vi "WPI_RobotDriveOpen6MotorWithVictor.vi"(0 "Rear Left Motor":T1=enum."PWM 2", 1 "Rear Left Motor Inverted":bool, 2 "Rear Right Motor Inverted":bool=TRUE, 5 "Rear Right Motor":T1, 7 "Front Left Motor":T1=enum."PWM 4", 9 "Front Right Motor":T1=enum."PWM 3", 11 "error in (no error)":errorcluster, 12 "Front Left Motor Inverted":bool, 13 "Front Right Motor Inverted":bool=TRUE) -> (4 "RobotDriveDevRef":T2={"DevStatus"={"status"=FALSE, "code"=0, "source"=""}, "Motors[]"=[], "Square Inputs"=FALSE, "Max Output"=1.0, "Isochronous"=FALSE}, 15 "error out":errorcluster)   [LabVIEW 2013]
doc: "Opens a reference to the robot drive for a four-motor robot using Victor motor controllers.\n\nThis software is licensed. Open the labview\\readme\\WPI Robotics Library Open Source License.txt file for more information."
uses:
  <vilib>/Rock Robotics/SystemInterfaces/DIO/FPGA_DIOPWMChannel.ctl
  <vilib>/Rock Robotics/WPI/RobotDrive/WPI_RobotDriveDevRef.ctl
  <vilib>/Rock Robotics/WPI/MotorControl/WPI_MotorControlDeviceRef.ctl
  <vilib>/Rock Robotics/SystemInterfaces/Typedef/FPGA_TypedefDigitalModule.ctl
  <vilib>/Rock Robotics/WPI/PWM/WPI_PWMDeadband.ctl
  <vilib>/Rock Robotics/WPI/CAN/Jaguar/SubVIs/WPI_CANJaguar_ControlMode.ctl
  <vilib>/Rock Robotics/WPI/PWM/WPI_PWMTransform_ConPane.ctl
  <vilib>/Rock Robotics/WPI/SafetyOutput/WPI_SafetyOutputConfigMenu.ctl
  <vilib>/Rock Robotics/WPI/MotorControl/WPI_MotorControlOpen Victor.vi
panel:
  in  "Mid Right Motor Inverted":bool=TRUE
  in  "Mid LeftMotor Inverted":bool
  in  "Mid Right Motor":T1=enum."PWM 5"
  in  "Mid Left Motor":T1=enum."PWM 6"
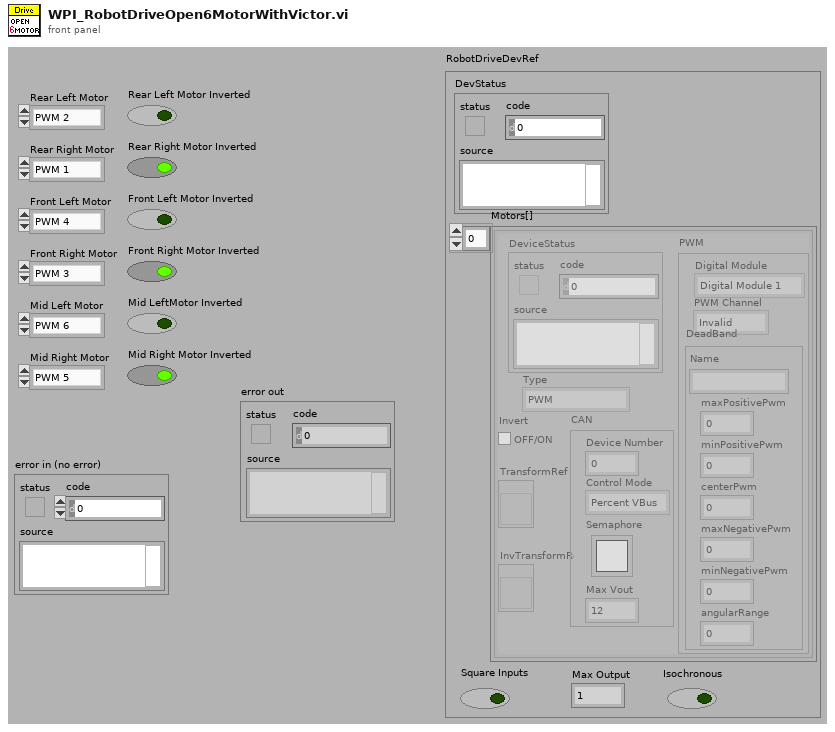
[diagram p1: front panel]
types:
  T1 = typedef "FPGA_DIOPWMChannel.ctl" = enum8{"PWM 1", "PWM 2", "PWM 3", "PWM 4", "PWM 5", "PWM 6", "PWM 7", "PWM 8", "PWM 9", "PWM 10", "Invalid"}
  T2 = typedef "WPI_RobotDriveDevRef.ctl" = cluster{"DevStatus":errorcluster, "Motors[]":T3[], "Square Inputs":bool, "Max Output":dbl, "Isochronous":bool}
  T3 = typedef "WPI_MotorControlDeviceRef.ctl" = cluster{"DeviceStatus":errorcluster, "Type":enum16{"PWM", "CAN"}, "PWM":cluster{"Digital Module":T4, "PWM Channel":T1, "DeadBand":T5}, "CAN":cluster{"Device Number":u8, "Control Mode":T6, "Semaphore":T7, "Max Vout":dbl}, "Invert":bool, "TransformRef":T8, "InvTransformRef":T8}
  T4 = typedef "FPGA_TypedefDigitalModule.ctl" = enum16{"Digital Module 1", "Digital Module 2"}
  T5 = typedef "WPI_PWMDeadband.ctl" = cluster{"Name":string, "maxPositivePwm":i32, "minPositivePwm":i32, "centerPwm":i32, "maxNegativePwm":i32, "minNegativePwm":i32, "angularRange":u16}
  T6 = typedef "WPI_CANJaguar_ControlMode.ctl" = enum8{"Percent VBus", "Current", "Speed", "Position", "Voltage"}
  T7 = typedef "Semaphore RefNum" = refnum<k1>
  T8 = typedef "WPI_PWMTransform_ConPane.ctl" = refnum<vi>
  T9 = typedef "WPI_SafetyOutputConfigMenu.ctl" = enum16{"Enable", "Disable"}
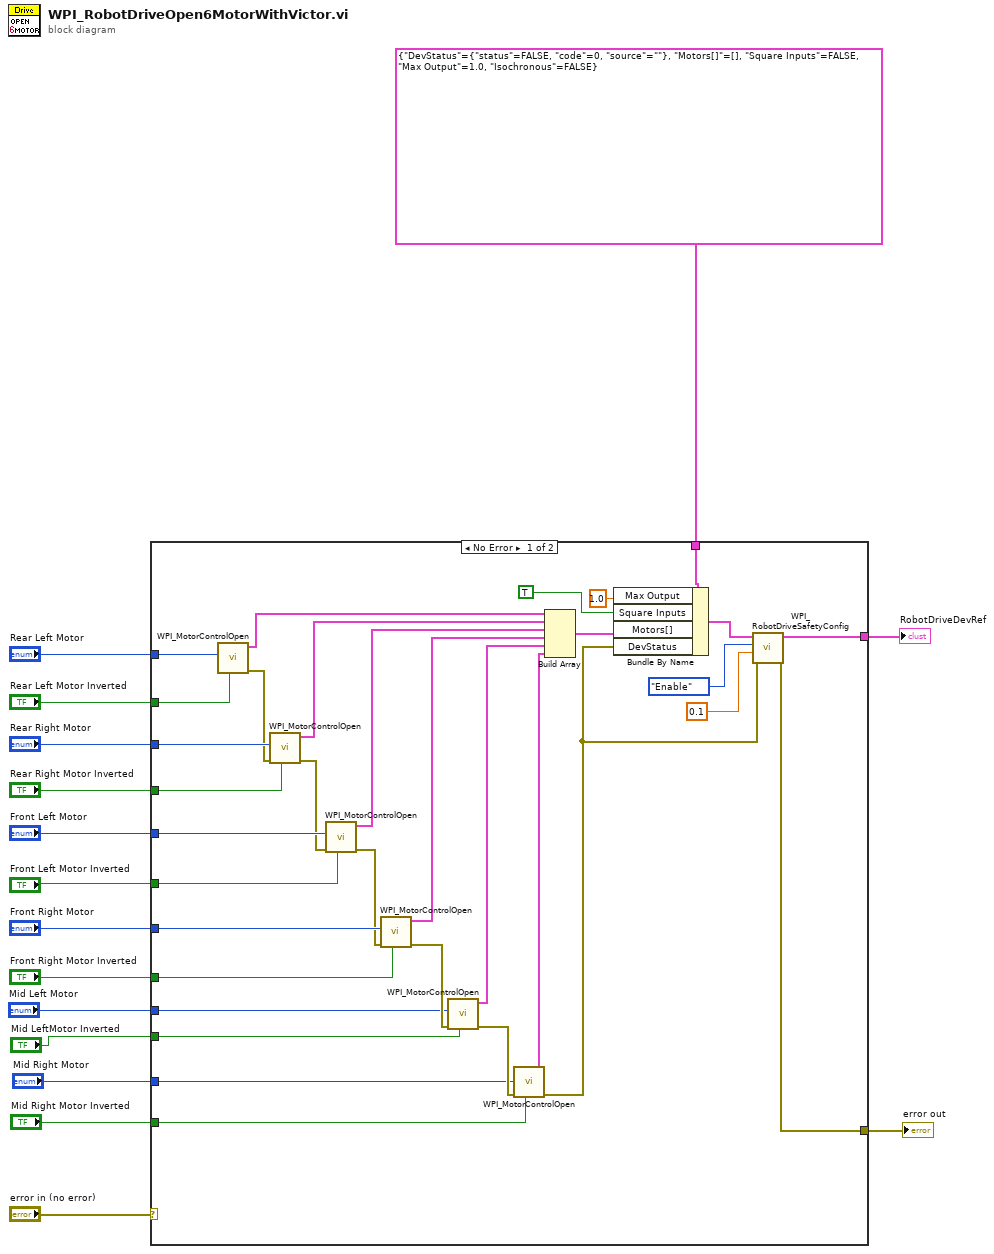
[diagram p0: block diagram]
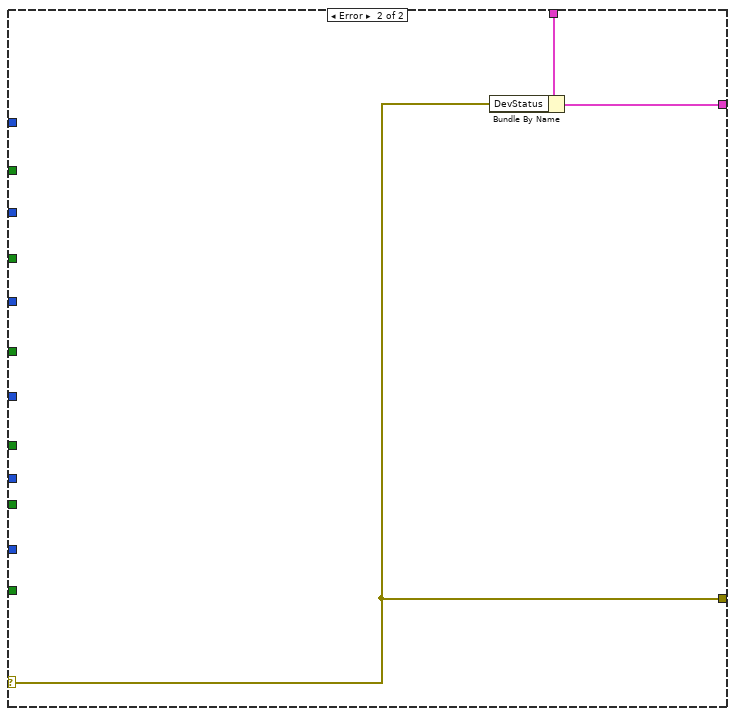
[diagram p2: hidden frame]
diagram:
  n1 = case shown="No Error" "error in (no error)" {
    selector: "error in (no error)" -> [_ w50]
    tunnel: [w28 w51] -> w16
    tunnel: T2 {"DevStatus"={"status"=FALSE, "code"=0, "source"=""}, "Motors[]"=[], "Square Inputs"=FALSE, "Max Output"=1.0, "Isochronous"=FALSE} ("RobotDriveDevRef") -> [w49 w52]
    tunnel: "Rear Left Motor" -> [w47 _]
    tunnel: "Front Right Motor" -> [w44 _]
    tunnel: "Front Left Motor" -> [w45 _]
    tunnel: "Rear Right Motor" -> [w46 _]
    tunnel: "Rear Left Motor Inverted" -> [w35 _]
    tunnel: "Rear Right Motor Inverted" -> [w34 _]
    tunnel: "Front Right Motor Inverted" -> [w32 _]
    tunnel: "Front Left Motor Inverted" -> [w33 _]
    tunnel: [w29 w50] -> w5
    tunnel: "Mid Left Motor" -> [w24 _]
    tunnel: "Mid LeftMotor Inverted" -> [w23 _]
    tunnel: "Mid Right Motor" -> [w20 _]
    tunnel: "Mid Right Motor Inverted" -> [w19 _]
    frame No Error {
      n2 = call-poly <vilib>:"WPI_MotorControlOpen.vi"("Invert"=w35, "PWM Channel"=w47) -> ("error out"=w37:errorcluster, "MotorControlDeviceRef"=w43:T3)  [unwired: 5 in, 3 out]
      n3 = call-poly <vilib>:"WPI_MotorControlOpen.vi"("Invert"=w34, "error in (no error)"=w37, "PWM Channel"=w46) -> ("error out"=w38:errorcluster, "MotorControlDeviceRef"=w42:T3)  [unwired: 4 in, 3 out]
      n4 = call-poly <vilib>:"WPI_MotorControlOpen.vi"("Invert"=w33, "error in (no error)"=w38, "PWM Channel"=w45) -> ("error out"=w39:errorcluster, "MotorControlDeviceRef"=w41:T3)  [unwired: 4 in, 3 out]
      n5 = call-poly <vilib>:"WPI_MotorControlOpen.vi"("Invert"=w32, "error in (no error)"=w39, "PWM Channel"=w44) -> ("error out"=w25:errorcluster, "MotorControlDeviceRef"=w40:T3)  [unwired: 4 in, 3 out]
      n6 = call-poly <vilib>:"WPI_MotorControlOpen.vi"("Invert"=w23, "error in (no error)"=w25, "PWM Channel"=w24) -> ("error out"=w21:errorcluster, "MotorControlDeviceRef"=w22:T3)  [unwired: 4 in, 3 out]
      n7 = call-poly <vilib>:"WPI_MotorControlOpen.vi"("Invert"=w19, "error in (no error)"=w21, "PWM Channel"=w20) -> ("error out"=w17:errorcluster, "MotorControlDeviceRef"=w18:T3)  [unwired: 4 in, 3 out]
      n8 = Build Array(w43, w42, w41, w40, w22, w18) -> (w36:T3[])
      n9 = Bundle By Name(cluster=w49, "Max Output"=1.0, "Square Inputs"=TRUE ("DestroyPWM?"), "Motors[]"=w36, "DevStatus"=w17) -> (w30:T2)
      n10 = call <vilib>:"WPI_RobotDriveSafetyConfig.vi"("error in (no error)"=w17, "timeout (s)"=0.1, "mode"=WPI_SafetyOutputConfigMenu."Enable", "RobotDriveDevRef"=w30) -> ("error out"=w29:errorcluster, "RobotDriveDevRef"=w28:T2)  [unwired: 6 out]
    }
    frame Error {
      n11 = Bundle By Name(cluster=w52, "DevStatus"=w50) -> (w51:T2)
    }
  }
  "RobotDriveDevRef" <- w16
  "error out" <- w5
